vi "ALONE_LKSHR_335.vi"(6 "Refresco(s)":dbl=0.25 caption="Elapsed Time (s)" format="%.2f", 8 "error in (no error)":errorcluster) -> (0 "Error Out":errorcluster, 7 "Enable":bool=TRUE)   [LabVIEW 2017]
uses:
  LAKESHORE/LS-335_Hardware_Module Control.ctl
  LAKESHORE/LS-335 SET PID.ctl
  <vilib>/Analysis/baseanly.llb/Mean (DBL).vi
  cRIO_ZNB_AMI_GLOBALES.vi
  <vilib>/gmath/NI_Gmath.lvlib
  <vilib>/Analysis/NI_AALBase.lvlib
panel:
  out "Output(%).":dbl format="%.2f"
  in  "Power Range":u16(ring) items=["Off", "Low (On)", "Medium", "High"]
  in  "Set":bool
  out "Temp Chart":dbl(graph)
  in  "Send":bool
  out "Array":dbl[](array[numeric])
  in  "q":i32=5 caption="Puntos, q" format="%#.0f"
  out "T Stable (T:yes)":bool caption="Stable"
  in  "sd max, %":dbl=5.0 caption="Desviacion max, %" format="%.1f"
  in  "Error max (K)":dbl=1.0 caption="Error" format="%.3f"
  out "Temperature Status":i32(ring) items=["TemperatureUnknown", "Stable", "Tracking", "Near"]
  out "Num 1":i32
  out "SetPoint(K).":dbl format="%.2f"
  in  "Setpoint T(K)":dbl format="%.2f"
  in  "Rate(K/min)":dbl format="%.2f"
  out "Temperatura(K).":dbl format="%.2f"
  out "ERROR":bool
  out "Date":string caption="asd"
  out "Time":string
  out "Refresh":bool
  in  "stop":bool
  # "Controlador Temperatura"
  # "STATUS"
  # "SETTINGS"
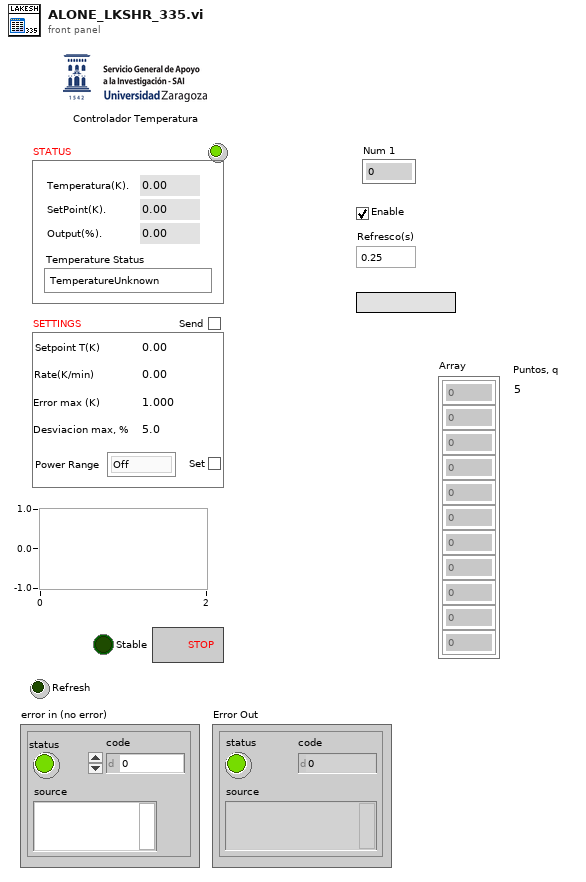
[diagram p1: front panel]
types:
  T1 = typedef "LS-335_Hardware_Module Control.ctl" = enum16{"INITIALIZE", "READ TEMPERATURE", "READ CONTROL DATA", "WRITE SETPOINT AND RATE", "WRITE PID AND POWER RANGE", "WRITE CONTROL PARAMETERS", "WRITE INPUT PARAMETERS", "SHUTDOWN"}
  T2 = typedef "LS-335 SET PID.ctl" = cluster{"Heater Output (1:1)":u16, "Gain (P) (50.0)":dbl, "Reset (I) (20.0)":dbl, "Rate (D) (0.0 %)":dbl, "Range (0:Off)":u16, "Manual Output (0.00 %)":dbl}
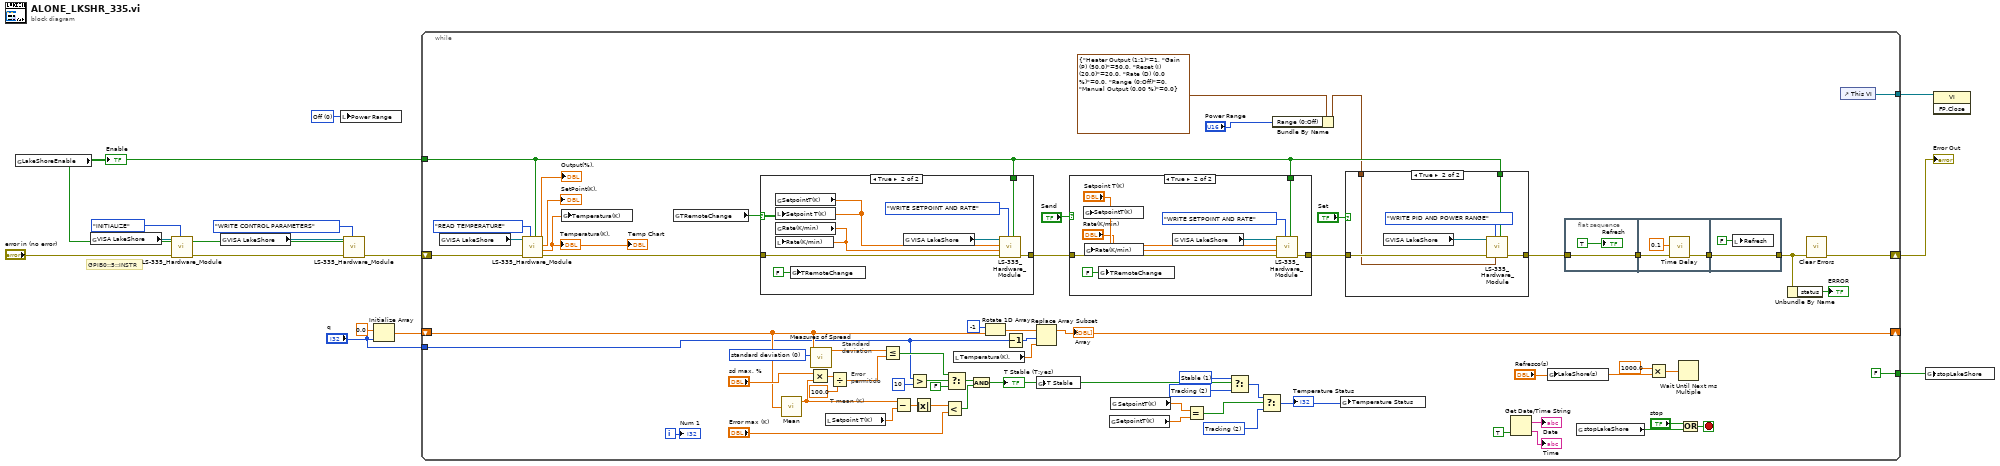
[diagram p0: block diagram]
diagram:
  w1 = u16 0 items=["Off", "Low (On)", "Medium", "High"] ("Range (0:Off)")
  # "GPIB0::5::INSTR"
  n1 = global read "cRIO_ZNB_AMI_GLOBALES.vi" "LakeShoreEnable"() -> (w7:bool)
  "Enable" <- w7
  n2 = global read "cRIO_ZNB_AMI_GLOBALES.vi" "VISA LakeShore"() -> (w11:refnum<visa-resource-name>)
  n3 = call "LS-335_Hardware_Module.vi"("Enable"=w7, "Command"=LS-335_Hardware_Module_Control."INITIALIZE", "error in (no error)"="error in (no error)", "VISA resource name"=w11) -> ("error out"=w8:errorcluster)  [unwired: 4 in, 3 out]
  n4 = global read "cRIO_ZNB_AMI_GLOBALES.vi" "VISA LakeShore"() -> (w5:refnum<visa-resource-name>)
  n5 = local write "Power Range"(w1) -> ()
  n6 = call "LS-335_Hardware_Module.vi"("Enable"=w7, "Command"=LS-335_Hardware_Module_Control."WRITE CONTROL PARAMETERS", "error in (no error)"=w8, "VISA resource name"=w5) -> ("error out"=w4:errorcluster)  [unwired: 4 in, 3 out]
  n7 = Initialize Array(0.0 ("element"), "q") -> (w3:dbl[])
  n8 = while {
    shift-right: [w70] -> w10
    shift-left: w4 -> [w69]
    tunnel: [FALSE ("stop")] -> w13
    tunnel: [w76] -> w15
    tunnel: w7 -> [w24]
    tunnel: "q" -> [w26]
    shift-right: [w30] -> _
    shift-left: w3 -> [w31]
    i -> [w66]
    stop <- w80 stop-if-true
    w44 = 0 items=["standard deviation", "range", "mean absolute deviation", "interquartile range"] ("type")
    w59 = 2 items=["TemperatureUnknown", "Stable", "Tracking", "Near"] ("Temperature Status")
    w58 = 2 items=["TemperatureUnknown", "Stable", "Tracking", "Near"] ("Temperature Status")
    w57 = 1 items=["TemperatureUnknown", "Stable", "Tracking", "Near"] ("Temperature Status")
    # "Error\npermitido"
    # "Standard\ndeviation"
    # "T mean (K)"
    n9 = global read "cRIO_ZNB_AMI_GLOBALES.vi" "VISA LakeShore"() -> (w56:refnum<visa-resource-name>)
    n10 = call "LS-335_Hardware_Module.vi"("Enable"=w24, "Command"=LS-335_Hardware_Module_Control."READ TEMPERATURE", "error in (no error)"=w69, "VISA resource name"=w56) -> ("error out"=w52:errorcluster, "Sensor Data"=w55:dbl, "Setpoint"=→"SetPoint(K).":dbl, "Output Value"=→"Output(%).":dbl)  [unwired: 4 in]
    "Temperatura(K)." <- w55
    "Temp Chart" <- w55
    n11 = global write "cRIO_ZNB_AMI_GLOBALES.vi" "Temperatura(K)"(w55) -> ()
    n12 = global read "cRIO_ZNB_AMI_GLOBALES.vi" "TRemoteChange"() -> (w53:bool)
    n13 = case shown="True" w53 {
      tunnel: w52 -> [w90 w94]
      tunnel: w24 -> [_ w96]
      tunnel: [w90 w95] -> w51
      frame False {
      }
      frame True {
        n14 = global read "cRIO_ZNB_AMI_GLOBALES.vi" "SetpointT(K)"() -> (w92:dbl)
        n15 = local write "Setpoint T(K)"(w92) -> ()
        n16 = global read "cRIO_ZNB_AMI_GLOBALES.vi" "Rate(K/min)"() -> (w91:dbl)
        n17 = local write "Rate(K/min)"(w91) -> ()
        n18 = global write "cRIO_ZNB_AMI_GLOBALES.vi" "TRemoteChange"(FALSE ("TRemoteChange")) -> ()
        n19 = global read "cRIO_ZNB_AMI_GLOBALES.vi" "VISA LakeShore"() -> (w98:refnum<visa-resource-name>)
        n20 = call "LS-335_Hardware_Module.vi"("Enable"=w96, "Command"=LS-335_Hardware_Module_Control."WRITE SETPOINT AND RATE", "error in (no error)"=w94, "Ramp Rate (0.0)"=w91, "Setpoint (0.0000)"=w92, "VISA resource name"=w98) -> ("error out"=w95:errorcluster)  [unwired: 2 in, 3 out]
      }
    }
    n21 = call-poly <vilib>:"Mean.vi"("X"=w31) -> ("mean"=w49:dbl)  [unwired: 1 out]
    n22 = Multiply(x="sd max, %", y=w49) -> (x*y=w39:dbl)
    n23 = call <vilib>:"Measures of Spread.vi"("type"=w44, "x array"=w31) -> ("spread value"=w35:dbl)  [unwired: 8 in, 1 out]
    n24 = local read "Setpoint T(K)"() -> (w28:dbl)
    n25 = Divide(x=w39, y=100.0) -> (x/y=w40:dbl)
    n26 = Less Or Equal?(x=w35, y=w40) -> (x <= y?=w37:bool)
    n27 = Subtract(x=w49, y=w28) -> (x-y=w41:dbl)
    n28 = Greater?(x=w26, y=10) -> (0:w36:bool)
    n29 = Absolute Value(x=w41) -> (abs(x)=w42:dbl)
    n30 = Less?(x=w42, y="Error max (K)") -> (x < y?=w43:bool)
    n31 = Select(t=w37, s=w36, f=FALSE ("TdownStable (T:yes)")) -> (s? t:f=w38:bool)
    n32 = local read "Temperatura(K)."() -> (w29:dbl)
    n33 = And(x=w38, y=w43) -> (x .and. y?=w27:bool)
    "T Stable (T:yes)" <- w27
    n34 = Rotate 1D Array(1:w31, 2:-1 ("n")) -> (0:w33:dbl[])
    n35 = Decrement(x=w26) -> (x-1=w32:i32)
    n36 = Replace Array Subset(array=w33, new element=w29, index=w32) -> (w30:dbl[])
    "Array" <- w30
    n37 = global write "cRIO_ZNB_AMI_GLOBALES.vi" "T Stable"(w27) -> ()
    n38 = case shown="True" "Send" {
      tunnel: w51 -> [w99 w103]
      tunnel: w24 -> [_ w105]
      tunnel: [w99 w104] -> w23
      frame False {
      }
      frame True {
        n39 = global write "cRIO_ZNB_AMI_GLOBALES.vi" "SetpointT(K)"("Setpoint T(K)") -> ()
        n40 = global write "cRIO_ZNB_AMI_GLOBALES.vi" "Rate(K/min)"("Rate(K/min)") -> ()
        n41 = global write "cRIO_ZNB_AMI_GLOBALES.vi" "TRemoteChange"(FALSE ("TRemoteChange")) -> ()
        n42 = global read "cRIO_ZNB_AMI_GLOBALES.vi" "VISA LakeShore"() -> (w107:refnum<visa-resource-name>)
        n43 = call "LS-335_Hardware_Module.vi"("Enable"=w105, "Command"=LS-335_Hardware_Module_Control."WRITE SETPOINT AND RATE", "error in (no error)"=w103, "Ramp Rate (0.0)"="Rate(K/min)", "Setpoint (0.0000)"="Setpoint T(K)", "VISA resource name"=w107) -> ("error out"=w104:errorcluster)  [unwired: 2 in, 3 out]
      }
    }
    n44 = global read "cRIO_ZNB_AMI_GLOBALES.vi" "SetpointT(K)"() -> (w64:dbl)
    n45 = global read "cRIO_ZNB_AMI_GLOBALES.vi" "SetpointT(K)"() -> (w65:dbl)
    n46 = Equal?(x=w65, y=w64) -> (x = y?=w62:bool)
    n47 = Select(t=w57, s=w27, f=w58) -> (s? t:f=w61:i32)
    n48 = Select(t=w61, s=w62, f=w59) -> (s? t:f=w60:i32)
    "Temperature Status" <- w60
    n49 = Bundle By Name(cluster=T2 {"Heater Output (1:1)"=1, "Gain (P) (50.0)"=50.0, "Reset (I) (20.0)"=20.0, "Rate (D) (0.0 %)"=0.0, "Range (0:Off)"=0, "Manual Output (0.00 %)"=0.0} ("PID Settings"), "Range (0:Off)"="Power Range") -> (w19:T2)
    n50 = global write "cRIO_ZNB_AMI_GLOBALES.vi" "Temperature Status"(w60) -> ()
    n51 = case shown="True" "Set" {
      tunnel: w23 -> [w83 w85]
      tunnel: w24 -> [_ w87]
      tunnel: [w83 w86] -> w22
      tunnel: w19 -> [_ w84]
      frame False {
      }
      frame True {
        n52 = global read "cRIO_ZNB_AMI_GLOBALES.vi" "VISA LakeShore"() -> (w89:refnum<visa-resource-name>)
        n53 = call "LS-335_Hardware_Module.vi"("Enable"=w87, "PID Settings"=w84, "Command"=LS-335_Hardware_Module_Control."WRITE PID AND POWER RANGE", "error in (no error)"=w85, "VISA resource name"=w89) -> ("error out"=w86:errorcluster)  [unwired: 3 in, 3 out]
      }
    }
    n54 = Get Date/Time String(want seconds? (F)=TRUE) -> (date string=→"Date":string, time string=→"Time":string)  [unwired: 2 in]
    n55 = global write "cRIO_ZNB_AMI_GLOBALES.vi" "LakeShore(s)"("Refresco(s)") -> ()
    n56 = flat-sequence {
      tunnel: w22 -> [w109]
      tunnel: [w109] -> w68
      tunnel: w68 -> [w111]
      tunnel: [w110] -> w67
      tunnel: [w113] -> w21
      tunnel: w67 -> [w113]
      frame #0 {
        "Refresh" <- TRUE ("Refresh")
      }
      frame #1 {
        n57 = call "Time Delay"("error in (no error)"=w111, "Delay Time (s)"=0.1) -> ("error out"=w110:errorcluster)  [unwired: 9 in]
      }
      frame #2 {
        n58 = local write "Refresh"(FALSE ("Refresh")) -> ()
      }
    }
    n59 = global read "cRIO_ZNB_AMI_GLOBALES.vi" "stopLakeShore"() -> (w75:bool)
    n60 = Multiply(x=1000.0, y="Refresco(s)") -> (x*y=w71:dbl)
    n61 = Wait Until Next ms Multiple(millisecond multiple=w71) -> ()  [unwired: 1 out]
    n62 = Or(x="stop", y=w75) -> (x .or. y?=w80:bool)
    n63 = Unbundle By Name(w21) -> ("status"=→"ERROR":bool)
    n64 = call <vilib>:"Clear Errors.vi"("error in (no error)"=w21) -> ("error out"=w70:errorcluster)  [unwired: 5 in, 1 out]
    n65 = control-ref of="This VI"() -> (w76:refnum<vi>)
    "Num 1" <- w66
  }
  "Error Out" <- w10
  n66 = global write "cRIO_ZNB_AMI_GLOBALES.vi" "stopLakeShore"(w13) -> ()
  n67 = invoke class="VI" method="FP.Close"(reference=w15) -> ()  [unwired: 2 in, 3 out]
